vi "Get ixon camera info.vi"() -> ()   [LabVIEW 2015]
uses:
  <userlib>/atmcd32d.llb/HSSpeed_type typedef.ctl
  <userlib>/atmcd32d.llb/AndorCapabilities typedef.ctl
panel:
  out "description":string
  out "InternalShutter?":i32
  out "Camera used":i32
  in  "Select camera number\n(starting with zero)":i32=1
  out "Camera handles":i32[](array[numeric])
  out "error out":errorcluster
  out "totalCameras":i32
  out "Preamp gains":sgl[](array[numeric])
  out "# y pixels":i32
  out "# x pixels":i32
  out "highest EM gain":i32
  out "lowest EM gain":i32
  out "camera serial #":i32
  out "Flex version #":u32
  out "PCB version #":u32
  out "head model":string
  out "VS speeds":sgl[](array[numeric])
  out "fastest recommended VS speed":sgl format="%.2f"
  out "Camera capabilities":T1
  in  "EM?":T2
  out "HS Speeds on each channel":sgl[][](array[numeric])
  out "bit depth each channel":i32[](array[numeric])
  out "#preamp gains":i32
  out "# amplifiers":i32
  out "#ADC channels":i32
  out "Return from Initialize":u32
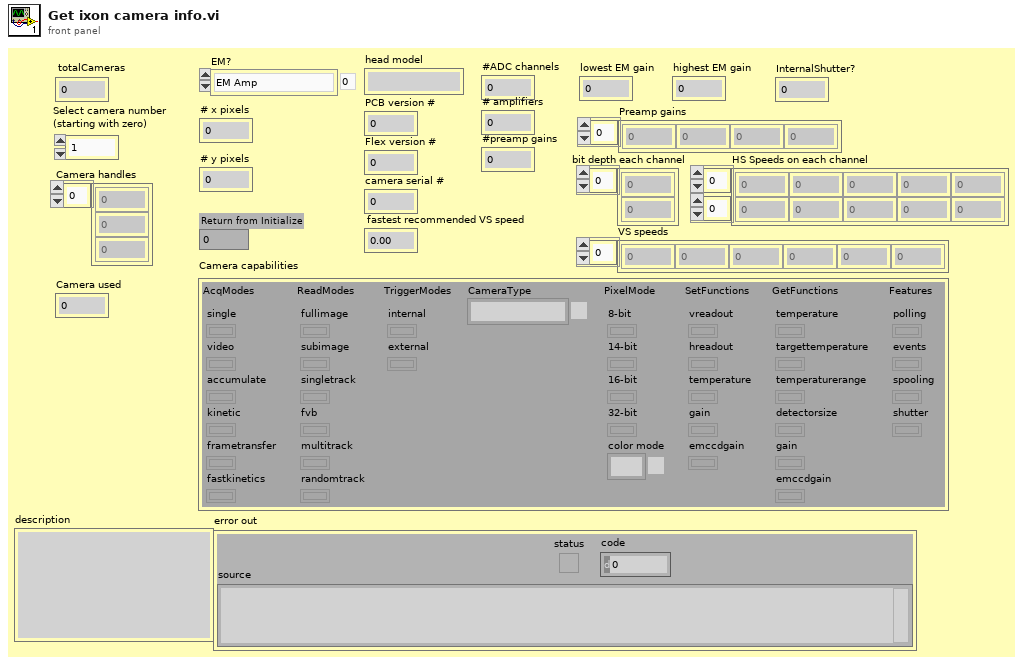
[diagram p1: front panel]
types:
  T1 = typedef "AndorCapabilities typedef.ctl" = cluster{"AcqModes":cluster{"single":bool, "video":bool, "accumulate":bool, "kinetic":bool, "frametransfer":bool, "fastkinetics":bool}, "ReadModes":cluster{"fullimage":bool, "subimage":bool, "singletrack":bool, "fvb":bool, "multitrack":bool, "randomtrack":bool}, "TriggerModes":cluster{"internal":bool, "external":bool}, "CameraType":enum32{"PDA", "iXon", "ICCD", "EMCCD", "CCD", "iStar", "third party camera", "iDus", "Newton", "Surcam", "USB ICCD", "Luca", "Reserved", "iKon", "InGaAs", "iVac", "Unprogrammed", "Clara", "USB iStar", "SimCam", "Neo", "iXon Ultra", "Volmos", "iVac Ultra"}, "PixelMode":cluster{"8-bit":bool, "14-bit":bool, "16-bit":bool, "32-bit":bool, "color mode":enum16{"Mono", "RGB", "CMY"}}, "SetFunctions":cluster{"vreadout":bool, "hreadout":bool, "temperature":bool, "gain":bool, "emccdgain":bool}, "GetFunctions":cluster{"temperature":bool, "targettemperature":bool, "temperaturerange":bool, "detectorsize":bool, "gain":bool, "emccdgain":bool}, "Features":cluster{"polling":bool, "events":bool, "spooling":bool, "shutter":bool}}
  T2 = typedef "HSSpeed_type typedef.ctl" = enum16{"EM Amp", "Conventional Amp"}
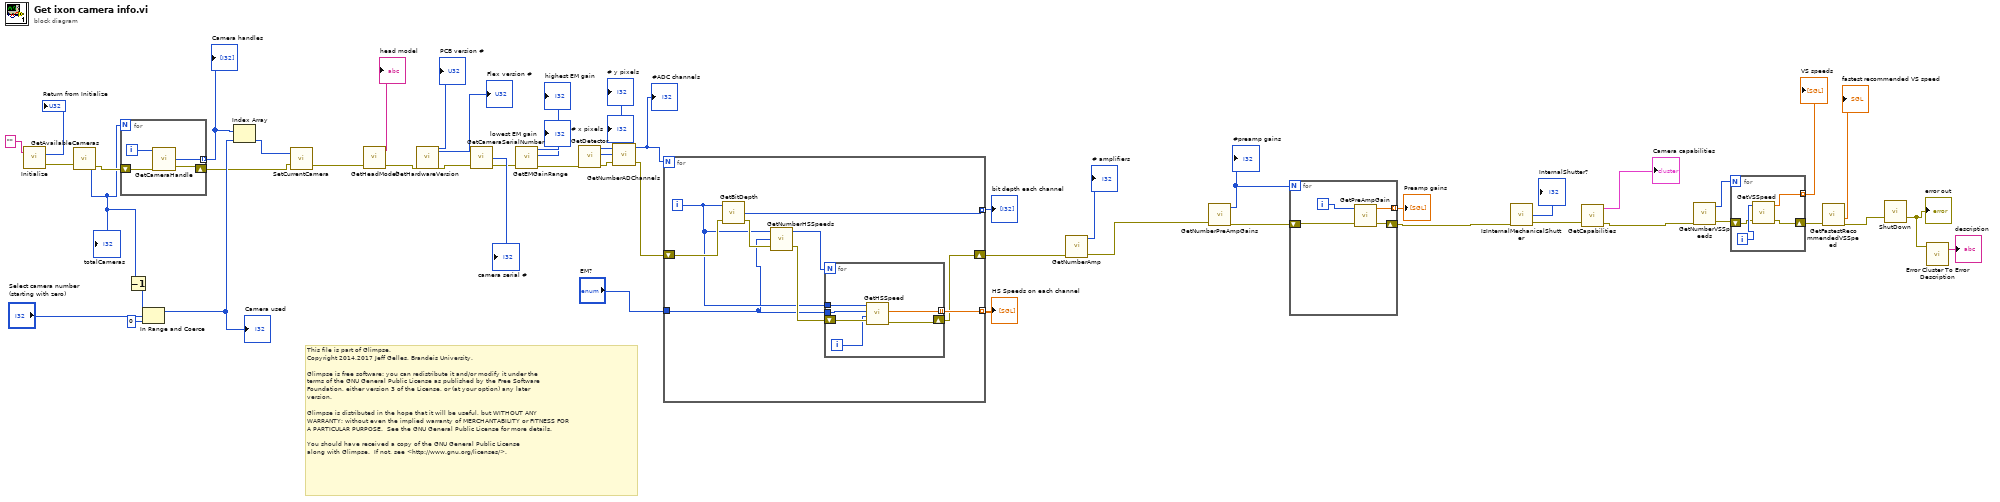
[diagram p0: block diagram]
diagram:
  # "This file is part of Glimpse. \nCopyright 2014,2017 Jeff Gelles, Brandeis University.    \n\nGlimpse is free software: you can redistribute it and/or modify it under the \nterms of the GNU General Public License as published by the Free Software \nFoundation, either version 3 of the License, or (at your option) any later \nversion.\n\nGlimpse is distributed in the hope that it will be useful, but WITHOUT ANY \nWARRANTY; without even the implied warranty of MERCHANTABILITY or FITNESS FOR \nA PARTICULAR PURPOSE.  See the GNU General Public License for more details.\n\nYou should have received a copy of the GNU General Public License\nalong with Glimpse.  If not, see <http://www.gnu.org/licenses/>."
  n1 = call <userlib>:"Initialize.vi"("directory (\"\")"="" ("directory (\"\")")) -> ("error out"=w16:errorcluster, "DLL error code"=→"Return from Initialize":u32)  [unwired: 1 in]
  n2 = call <userlib>:"GetAvailableCameras.vi"("error in (no error)"=w16) -> ("error out"=w15:errorcluster, "totalCameras"=w12:i32)  [unwired: 2 in, 1 out]
  "totalCameras" <- w12
  n3 = for {
    N: w12 -> [_]
    shift-right: [w53] -> w8
    shift-left: w15 -> [w54]
    tunnel: [w51] -> w14 mode=indexing
    i -> [w52]
    n4 = call <userlib>:"GetCameraHandle.vi"("error in (no error)"=w54, "cameraIndex"=w52) -> ("error out"=w53:errorcluster, "cameraHandle"=w51:i32)  [unwired: 1 in, 1 out]
  }
  "Camera handles" <- w14
  n5 = Decrement(x=w12) -> (x-1=w6:i32)
  n6 = In Range and Coerce(upper limit=w6, x="Select camera number\n(starting with zero)", lower limit=0) -> (coerced(x)=w10:i32)  [unwired: 1 out]
  "Camera used" <- w10
  n7 = Index Array(array=w14, index=w10) -> (element=w7:i32)
  n8 = call <userlib>:"SetCurrentCamera.vi"("error in (no error)"=w8, "cameraHandle"=w7) -> ("error out"=w9:errorcluster)  [unwired: 1 out]
  n9 = call <userlib>:"GetHeadModel.vi"("error in (no error)"=w9) -> ("error out"=w23:errorcluster, "model"=→"head model":string)  [unwired: 2 in, 1 out]
  n10 = call <userlib>:"GetHardwareVersion.vi"("error in (no error)"=w23) -> ("PCB"=→"PCB version #":u32, "Flex"=→"Flex version #":u32, "error out"=w22:errorcluster)  [unwired: 19 in, 5 out]
  n11 = call <userlib>:"GetCameraSerialNumber.vi"("error in (no error)"=w22) -> ("error out"=w21:errorcluster, "number"=→"camera serial #":i32)  [unwired: 2 in, 1 out]
  n12 = call <userlib>:"GetEMGainRange.vi"("error in (no error)"=w21) -> ("error out"=w20:errorcluster, "high"=→"highest EM gain":i32, "low"=→"lowest EM gain":i32)  [unwired: 3 in, 1 out]
  n13 = call <userlib>:"GetDetector.vi"("error in (no error)"=w20) -> ("error out"=w26:errorcluster, "ypixels"=→"# y pixels":i32, "xpixels"=→"# x pixels":i32)  [unwired: 3 in, 1 out]
  n14 = call <userlib>:"GetNumberADChannels.vi"("error in (no error)"=w26) -> ("error out"=w46:errorcluster, "number"=w47:i32)  [unwired: 2 in, 1 out]
  "#ADC channels" <- w47
  n15 = for {
    N: w47 -> [_]
    shift-right: [w57] -> w44
    shift-left: w46 -> [w63]
    tunnel: [w62] -> w45 mode=indexing
    tunnel: [w58] -> w42 mode=indexing
    tunnel: "EM?" -> [w55]
    i -> [w56]
    n16 = call <userlib>:"GetBitDepth.vi"("error in (no error)"=w63, "channel"=w56) -> ("error out"=w61:errorcluster, "depth"=w62:i32)  [unwired: 1 in, 1 out]
    n17 = call <userlib>:"GetNumberHSSpeeds.vi"("error in (no error)"=w61, "type"=w55, "channel"=w56) -> ("error out"=w60:errorcluster, "number"=w59:i32)  [unwired: 1 out]
    n18 = for {
      N: w59 -> [_]
      shift-right: [w67] -> w57
      shift-left: w60 -> [w69]
      tunnel: [w68] -> w58 mode=indexing
      tunnel: w56 -> [w66]
      tunnel: w55 -> [w65]
      i -> [w64]
      n19 = call <userlib>:"GetHSSpeed.vi"("error in (no error)"=w69, "index"=w64, "type"=w65, "channel"=w66) -> ("error out"=w67:errorcluster, "speed"=w68:sgl)  [unwired: 1 in, 1 out]
    }
  }
  "bit depth each channel" <- w45
  "HS Speeds on each channel" <- w42
  n20 = call <userlib>:"GetNumberAmp.vi"("error in (no error)"=w44) -> ("error out"=w43:errorcluster, "number"=→"# amplifiers":i32)  [unwired: 2 in, 1 out]
  n21 = call <userlib>:"GetNumberPreAmpGains.vi"("error in (no error)"=w43) -> ("error out"=w18:errorcluster, "number"=w19:i32)  [unwired: 2 in, 1 out]
  "#preamp gains" <- w19
  n22 = for {
    N: w19 -> [_]
    shift-right: [w72] -> w5
    shift-left: w18 -> [w71]
    tunnel: [w70] -> w17 mode=indexing
    i -> [w73]
    n23 = call <userlib>:"GetPreAmpGain.vi"("error in (no error)"=w71, "index"=w73) -> ("error out"=w72:errorcluster, "gain"=w70:sgl)  [unwired: 1 in, 1 out]
  }
  "Preamp gains" <- w17
  n24 = call <userlib>:"IsInternalMechanicalShutter.vi"("error in (no error)"=w5) -> ("error out"=w4:errorcluster, "InternalShutter"=→"InternalShutter?":i32)  [unwired: 2 in, 1 out]
  n25 = call <userlib>:"GetCapabilities.vi"("error in (no error)"=w4) -> ("error out"=w34:errorcluster, "caps"=→"Camera capabilities":T1)  [unwired: 2 in, 1 out]
  n26 = call <userlib>:"GetNumberVSSpeeds.vi"("error in (no error)"=w34) -> ("error out"=w35:errorcluster, "number"=w33:i32)  [unwired: 2 in, 1 out]
  n27 = for {
    N: w33 -> [_]
    tunnel: [w77] -> w37 mode=indexing
    shift-right: [w76] -> w36
    shift-left: w35 -> [w74]
    i -> [w75]
    n28 = call <userlib>:"GetVSSpeed.vi"("error in (no error)"=w74, "index"=w75) -> ("error out"=w76:errorcluster, "speed"=w77:sgl)  [unwired: 1 in, 1 out]
  }
  "VS speeds" <- w37
  n29 = call <userlib>:"GetFastestRecommendedVSSpeed.vi"("error in (no error)"=w36) -> ("error out"=w38:errorcluster, "speed"=→"fastest recommended VS speed":sgl)  [unwired: 3 in, 2 out]
  n30 = call <userlib>:"ShutDown.vi"("error in (no error)"=w38) -> ("error out"=w2:errorcluster)  [unwired: 1 in, 1 out]
  "error out" <- w2
  n31 = call <userlib>:"Error Cluster To Error Description.vi"("error cluster"=w2) -> ("description"=→"description":string)  [unwired: 3 in, 1 out]
